vi "G#Object_GetClassPath.vi"(0 "reference in":refnum<class "G#Object.lvclass">, 5 "error in (no error)":errorcluster) -> (14 "reference out":refnum<class "G#Object.lvclass">, 15 "class path":path, 19 "error out":errorcluster)   [LabVIEW 2017, in "G#Object.lvclass"]
doc: "Returns the path to the lvclass file."
uses:
  G#Object.lvclass
  <vilib>/Utility/error.llb/Error Cluster From Error Code.vi
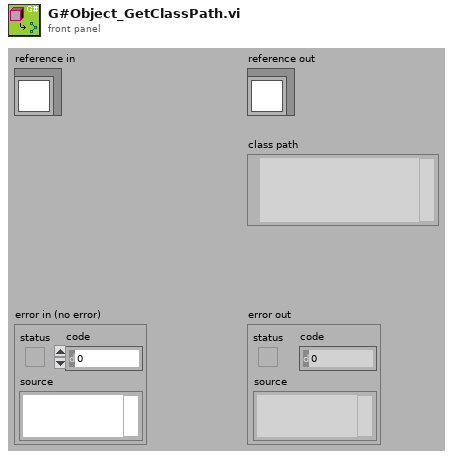
[diagram p1: front panel]
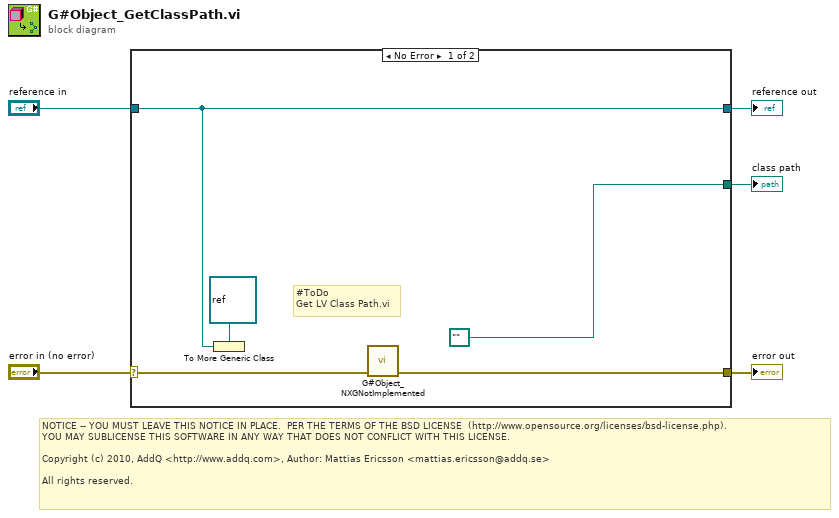
[diagram p0: block diagram]
diagram:
  # "NOTICE -- YOU MUST LEAVE THIS NOTICE IN PLACE.  PER THE TERMS OF THE BSD LICENSE  (http://www.opensource.org/licenses/bsd-license.php).\nYOU MAY SUBLICENSE THIS SOFTWARE IN ANY WAY THAT DOES NOT CONFLICT WITH THIS LICENSE.\n\nCopyright (c) 2010, AddQ <http://www.addq.com>, Author: Mattias Ericsson <mattias.ericsson@addq.se>\n\nAll rights reserved."
  n1 = case shown="No Error" "error in (no error)" {
    selector: "error in (no error)" -> [w7 w12]
    tunnel: [w6 w12] -> w4
    tunnel: [w9 w11] -> w2
    tunnel: "reference in" -> [w9 w11]
    tunnel: [path "" ("class path") _] -> w1
    frame No Error {
      # "#ToDo\nGet LV Class Path.vi"
      n2 = To More Generic Class(target class=refnum<class> refnum ("object"), reference=w9) -> ()  [unwired: 1 out]
      n3 = call "G#Object_NXGNotImplemented.vi"("error in"=w7) -> ("error out"=w6:errorcluster)  [unwired: 18 in]
    }
    frame Error {
    }
  }
  "error out" <- w4
  "reference out" <- w2
  "class path" <- w1
